vi "Signal Processing - BelowThreshold.vi"(10 "Threshold":dbl, 11 "signal in":waveform(dbl)) -> (3 "Output":i32)   [LabVIEW 2010, in "Core SubVIs.lvlib"]
uses:
  Core SubVIs.lvlib
  <vilib>/Waveform/WDTOps.llb/WDT Waveform to XY Pairs DBL.vi
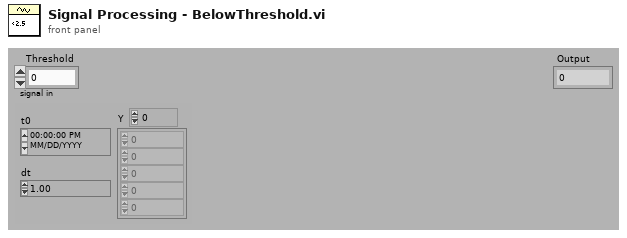
[diagram p1: front panel]
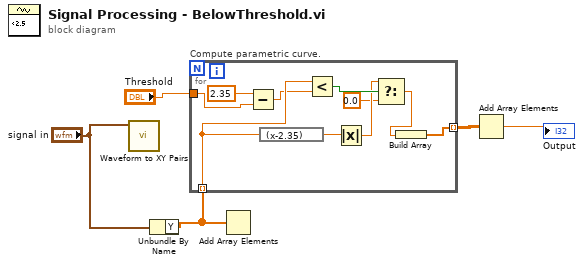
[diagram p0: block diagram]
diagram:
  n1 = call-poly <vilib>:"Waveform to XY Pairs.vi"("waveform in"="signal in") -> ()  [unwired: 8 in, 3 out]
  n2 = Unbundle By Name("signal in") -> ("Y"=w3:dbl[])
  n3 = for "Compute parametric curve." {
    tunnel: [w15] -> w5 mode=indexing
    tunnel: w3 -> [w14] mode=indexing
    tunnel: "Threshold" -> [w6]
    n4 = Subtract(x=2.35, y=w6) -> (x-y=w13:dbl)
    n5 = expression code="(x-2.35)"(w14) -> (w12:dbl)
    n6 = Less?(x=w14, y=w13) -> (x < y?=w11:bool)
    n7 = Absolute Value(x=w12) -> (abs(x)=w10:dbl)
    n8 = Select(t=w10, s=w11, f=0.0) -> (s? t:f=w8:dbl)
    n9 = Build Array(w8) -> (w15:dbl[])
  }
  n10 = Add Array Elements(numeric array=w3) -> ()  [unwired: 1 out]
  n11 = Add Array Elements(numeric array=w5) -> (sum=→"Output":dbl)
